vi "Float32 Create.vi"(8 "error in (no error)":errorcluster, 11 "SGL in":sgl) -> (0 "error out":errorcluster, 3 "Float32 DVR out":refnum<data-value>)   [LabVIEW 2012, in "MDSplus.lvlib"]
uses:
  <vilib>/MDSplus/Library/MDSplus.lvlib
  <vilib>/MDSplus/Classes/Data_Class/Scalar_Class/Float32_Class/Float32.lvclass
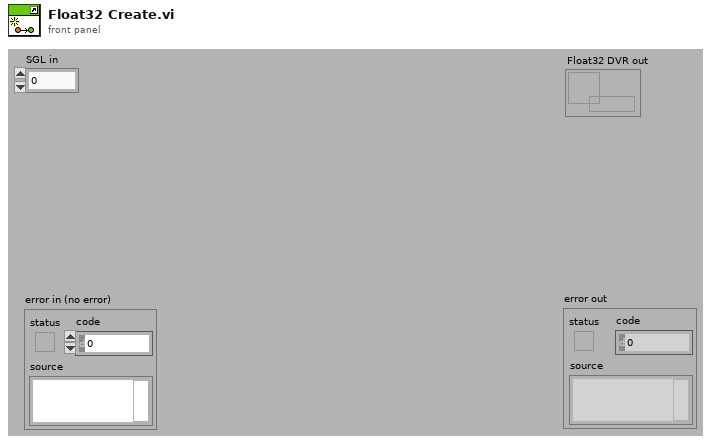
[diagram p1: front panel]
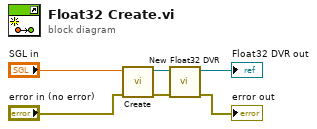
[diagram p0: block diagram]
diagram:
  n1 = call <vilib>:"Create.vi"("error in (no error)"="error in (no error)", "SGL in"="SGL in") -> ("error out"=w3:errorcluster, "Float32 out"=w4:refnum<class "Float32.lvclass">)  [unwired: 8 in]
  n2 = call <vilib>:"New Float32 DVR.vi"("error in (no error)"=w3, "Float32 in"=w4) -> ("error out"=→"error out":errorcluster, "Float32 DVR out"=→"Float32 DVR out":refnum<data-value>)  [unwired: 8 in]
